vi "Get Result.vi"(6 "Last request":bool, 8 "error in (no error)":errorcluster, 11 "Instrument Recorder in":refnum<class "Instrument Actor.lvclass">) -> (0 "error out":errorcluster, 2 "Result":refnum<class "Acquired Result.lvclass">, 3 "Instrument Recorder out":refnum<class "Instrument Actor.lvclass">)   [LabVIEW 2016, in "Instrument Actor.lvclass"]
uses:
  Instrument Actor.lvclass
  Results/Acquired Result/Acquired Result.lvclass
  Instrument Actor.lvclass/Instrument Actor.ctl
  Read Instrument driver.vi
  Write Instrument driver.vi
  NHMFL_Core/Libraries/Instruments/Instrument Driver/Instrument Driver.lvclass
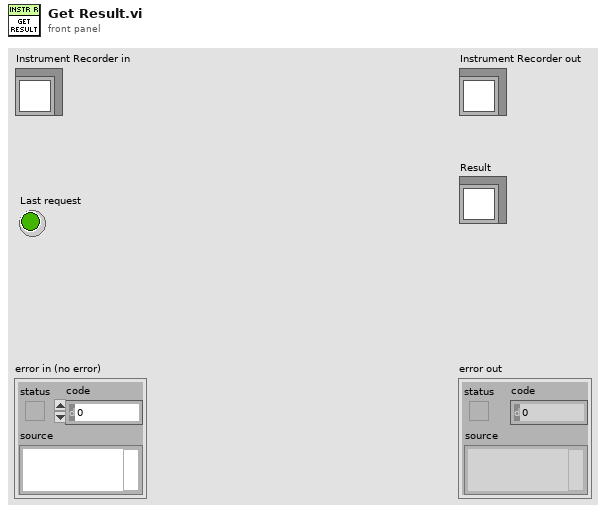
[diagram p1: front panel]
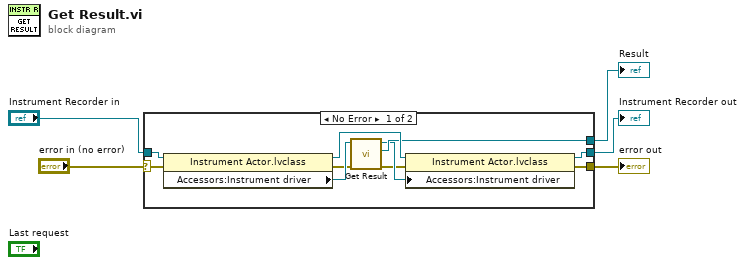
[diagram p0: block diagram]
diagram:
  n1 = case shown="No Error" "error in (no error)" {
    selector: "error in (no error)" -> [w8 w17]
    tunnel: [w6 w17] -> w4
    tunnel: [w11 w16] -> w2
    tunnel: "Instrument Recorder in" -> [w15 w16]
    tunnel: [w12 _] -> w1
    frame No Error {
      n2 = property class="Instrument Actor.lvclass"(reference=w15, error in=w8) -> (reference out=w14:refnum<class "Instrument Actor.lvclass">, error out=w9:errorcluster, "Accessors:Instrument driver"=w13:refnum<class "Instrument Driver.lvclass">)
      n3 = call-dynamic "Get Result.vi"("error in (no error)"=w9, "Instrument Driver in"=w13) -> ("error out"=w7:errorcluster, "Result"=w12:refnum<class "Acquired Result.lvclass">, "Instrument Driver out"=w10:refnum<class "Instrument Driver.lvclass">)  [unwired: 7 in]
      n4 = property class="Instrument Actor.lvclass"(reference=w14, error in=w7, "Accessors:Instrument driver"=w10) -> (reference out=w11:refnum<class "Instrument Actor.lvclass">, error out=w6:errorcluster)
    }
    frame Error {
    }
  }
  "error out" <- w4
  "Instrument Recorder out" <- w2
  "Result" <- w1
